vi "writeToXML.vi"(8 "error in (no error)":errorcluster, 10 "Class Label":string="GWTargetPositionParameters", 11 "GWTargetPositionParameters in":refnum<class "GWTargetPositionParameters.lvclass">) -> (0 "error out":errorcluster, 2 "outputXMLString":string="<>\n  <gTargTime>0</gTargTime>\n  <trackID>0</trackID>\n  <xPosition_mm>0</xPosition_mm>\n  <yPosition_mm>0</yPosition_mm>\n</>", 3 "GWTargetPositionParameters out":refnum<class "GWTargetPositionParameters.lvclass">)   [LabVIEW 2014, in "TCSDataDefinitions.lvlib" / "TCSGuiderStatus.lvlib" / "GWTargetPositionParameters.lvclass"]
uses:
  GWTargetPositionParameters.lvclass
  <userlib>/Common/UnitsAndXML/FlattenItemWithUnitToXML/FlattenLengthToXML/LengthUnit.ctl
  GWTargetPositionParameters.lvclass/GWTargetPositionParameters.ctl
  <userlib>/Common/UnitsAndXML/UnitsAndXML.lvlib
  <userlib>/Common/XML/XMLGenerator/XMLGenerator.lvclass
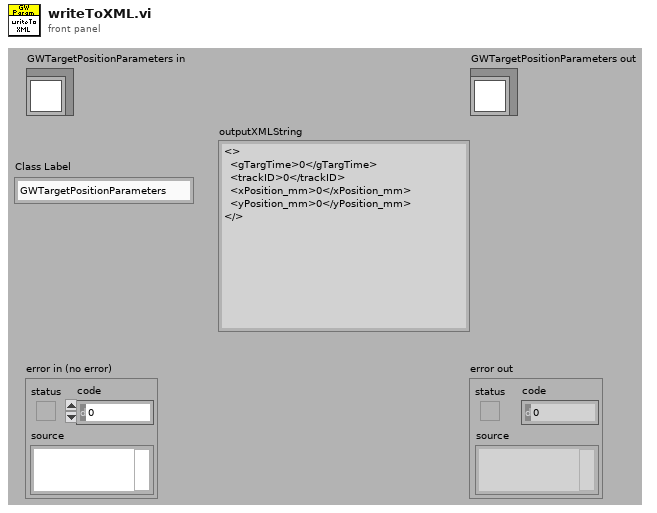
[diagram p1: front panel]
types:
  T1 = typedef "UnitsAndXML.lvlib/LengthUnit.ctl" = enum16{"m", "Angstrom", "AU", "chain", "cm", "cubit", "fathom", "fermi", "ft", "furlong", "hubble", "in", "ly", "mi", "mm", "rod", "um", "yd"}
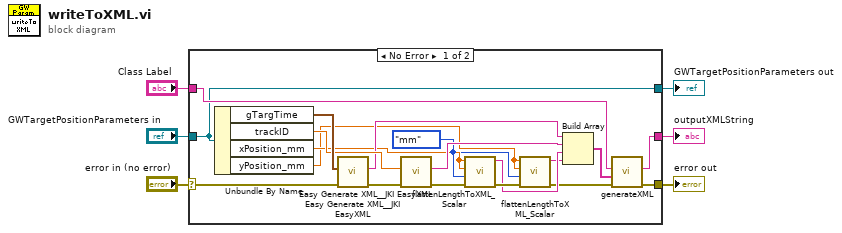
[diagram p0: block diagram]
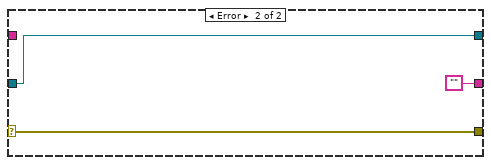
[diagram p2: hidden frame]
diagram:
  n1 = case shown="No Error" "error in (no error)" {
    selector: "error in (no error)" -> [w17 w28]
    tunnel: [w16 w28] -> w5
    tunnel: [w8 w27] -> w3
    tunnel: "GWTargetPositionParameters in" -> [w8 w27]
    tunnel: [w18 ""] -> w2
    tunnel: "Class Label" -> [w19 _]
    frame No Error {
      w12 = LengthUnit."mm" ("lengthUnitInXML")
      n2 = Unbundle By Name(w8) -> ("gTargTime"=w24:timestamp, "trackID"=w23:dbl, "xPosition_mm"=w13:dbl[unit], "yPosition_mm"=w11:dbl[unit])
      n3 = call <vilib>:"Easy Generate XML__JKI EasyXML.vi"("error in (no error)"=w17, "LabVIEW Data"=w24) -> ("error out"=w25:errorcluster, "XML String"=w21:string)  [unwired: 8 in]
      n4 = call <vilib>:"Easy Generate XML__JKI EasyXML.vi"("error in (no error)"=w25, "LabVIEW Data"=w23) -> ("error out"=w14:errorcluster, "XML String"=w22:string)  [unwired: 8 in]
      n5 = call <userlib>:"flattenLengthToXML_Scalar.vi"("error in (no error)"=w14, "lengthUnitInXML"=w12, "lengthAgain"=w13, "length"=w13) -> ("error out"=w15:errorcluster, "xmlString"=w10:string)  [unwired: 6 in]
      n6 = call <userlib>:"flattenLengthToXML_Scalar.vi"("error in (no error)"=w15, "lengthUnitInXML"=w12, "lengthAgain"=w11, "length"=w11) -> ("error out"=w7:errorcluster, "xmlString"=w9:string)  [unwired: 6 in]
      n7 = Build Array(w21, w22, w10, w9) -> (w20:string[])
      n8 = call <userlib>:"generateXML.vi"("error in"=w7, "childrenXML"=w20, "elementName"=w19) -> ("error out"=w16:errorcluster, "XML out"=w18:string)  [unwired: 6 in, 1 out]
    }
    frame Error {
    }
  }
  "error out" <- w5
  "GWTargetPositionParameters out" <- w3
  "outputXMLString" <- w2
